vi "AFT Filter Signal and Update Coefficients (Real, PtByPt).vi"(6 "step size":dbl=-1.0, 7 "reset? (F)":bool, 8 "error in (no error)":errorcluster, 9 "d(n)":dbl, 10 "x(n)":dbl, 11 "adaptive filter in":refnum<k20>) -> (0 "error out":errorcluster, 1 "e(n)":dbl, 2 "y(n)":dbl, 3 "adaptive filter out":refnum<k20>)   [LabVIEW 2017, in "NI_AdaptiveFilter.lvlib"]
doc: "Filters an input signal with an adaptive filter and updates the coefficients of the adaptive filter iteratively. You must use the least mean squares (LMS) or recursive least squares (RLS) algorithms to create the adaptive filter. Wire data to the <B>x(n)</B> and <B>d(n)</B> inputs to determine the polymorphic instance to use or manually select the instance. The data type of the adaptive filter that you wire to the <B>adaptive filter in</B> input must match the instance of the AFT Filter Signal and Update Coefficients VI."
uses:
  <vilib>/addons/Adaptive Filters/NI_AdaptiveFilter.lvlib
  <resource>/AdaptiveFilters.dll
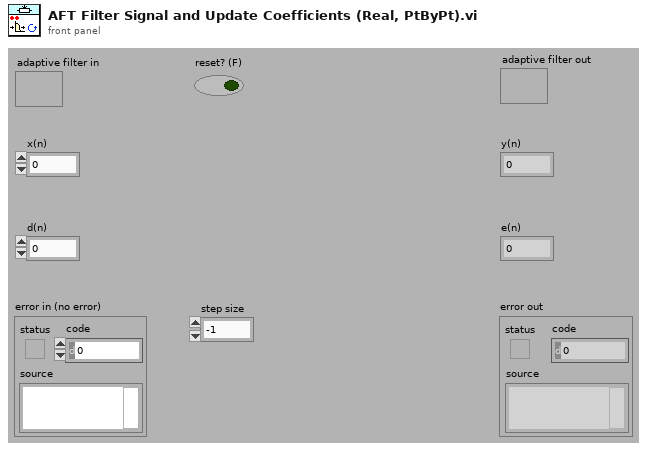
[diagram p1: front panel]
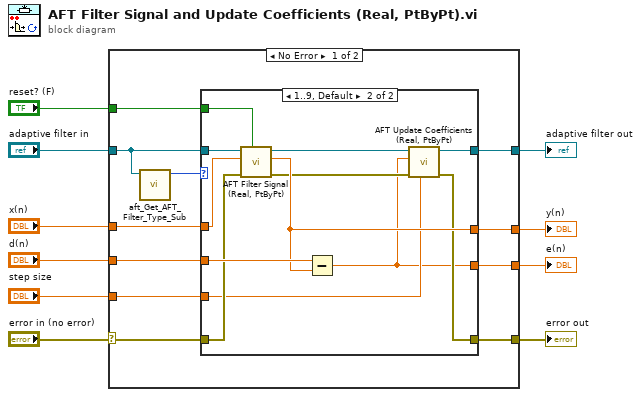
[diagram p0: block diagram]
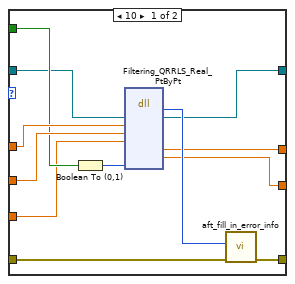
[diagram p2: hidden frame]
diagram:
  n1 = case shown="No Error" "error in (no error)" {
    selector: "error in (no error)" -> [w17 w47]
    tunnel: [w16 w47] -> w10
    tunnel: "adaptive filter in" -> [w12 w46]
    tunnel: "x(n)" -> [w21 _]
    tunnel: "d(n)" -> [w20 _]
    tunnel: [w18 w46] -> w6
    tunnel: "step size" -> [w15 _]
    tunnel: [w19 _] -> w4
    tunnel: [w13 _] -> w3
    tunnel: "reset? (F)" -> [w14 _]
    frame No Error {
      n2 = call <vilib>:"aft_Get_AFT_Filter_Type_Sub.vi"("adaptive filter in"=w12) -> ("type"=w11:i32)  [unwired: 9 out]
      n3 = case shown="1..9, Default" w11 {
        tunnel: w21 -> [w30 w45]
        tunnel: w20 -> [w29 w44]
        tunnel: [w28 w43] -> w19
        tunnel: w12 -> [w23 w41]
        tunnel: [w22 w40] -> w18
        tunnel: w17 -> [w32 w39]
        tunnel: [w31 w38] -> w16
        tunnel: w15 -> [w24 w36]
        tunnel: w14 -> [w26 w35]
        tunnel: [w27 w34] -> w13
        frame 10 {
          n4 = Boolean To (0,1)(Boolean=w26) -> (0, 1=w25:i16)
          n5 = dll-call lib="C:/Program Files/National Instruments/LabVIEW 2017/resource/AdaptiveFilters.dll" fn="Filtering_QRRLS_Real_PtByPt" ("Complex Data Initialization")("pSession"=w23, "x"=w30, "d"=w29, "mu"=w24, "reset"=w25) -> ("err"=w33:i32, "pSession"=w22:refnum<k20>, "y"=w28:dbl, "e"=w27:dbl)  [unwired: 7 in, 4 out]
          n6 = call <vilib>:"aft_fill_in_error_info.vi"("error in"=w32, "status code"=w33) -> ("error out"=w31:errorcluster)  [unwired: 2 in, 7 out]
        }
        frame 1..9, Default {
          n7 = call <vilib>:"AFT Filter Signal (Real, PtByPt).vi"("reset? (F)"=w35, "error in (no error)"=w39, "x(n)"=w45, "adaptive filter in"=w41) -> ("error out"=w37:errorcluster, "y(n)"=w43:dbl, "adaptive filter out"=w42:refnum<k20>)  [unwired: 5 out]
          n8 = Subtract(x=w44, y=w43) -> (x-y=w34:dbl)
          n9 = call <vilib>:"AFT Update Coefficients (Real, PtByPt).vi"("step size"=w36, "error in (no error)"=w37, "e(n)"=w34, "adaptive filter in"=w42) -> ("error out"=w38:errorcluster, "adaptive filter out"=w40:refnum<k20>)  [unwired: 6 out]
        }
      }
    }
    frame Error {
    }
  }
  "error out" <- w10
  "y(n)" <- w4
  "e(n)" <- w3
  "adaptive filter out" <- w6
